vi "finish5PreparePassGamePlay.vi"(8 "error in (no error)":errorcluster, 9 "last_command":T1, 10 "Game":refnum<class "Game.lvclass">, 11 "5PreparePassGamePlay in":refnum<class "5PreparePassGamePlay.lvclass">) -> (0 "error out":errorcluster, 2 "result":bool, 3 "5PreparePassGamePlay out":refnum<class "5PreparePassGamePlay.lvclass">)   [LabVIEW 2020, in "5PreparePassGamePlay.lvclass"]
uses:
  5PreparePassGamePlay.lvclass
  Game_class/Game.lvclass
  Referee_class/command_interpreted.ctl
  Game_class/Game.lvclass/Game.ctl
  Referee_class/Referee.lvclass/Referee.ctl
  Referee_class/Read command_interpreted.vi
  Game_class/Read Referee.vi
  Game_class/Read TimeRef.vi
  Referee_class/Referee.lvclass
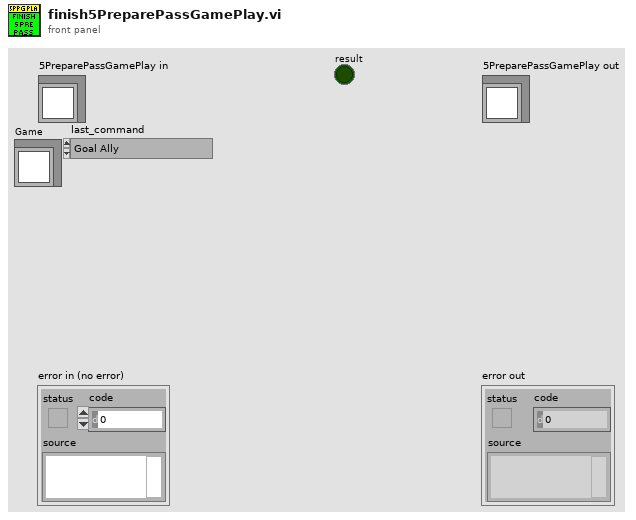
[diagram p1: front panel]
types:
  T1 = typedef "command_interpreted.ctl" = enum16{"Goal Ally", "Goal Enemy", "Ball Placement Enemy", "Ball Placement Ally", "Normal Half Time", "Extra Time  Break", "Extra Half Time", "None", "Post Game", "PKA Normal Start", "Prepare Kickoff Ally", "PKE Normal Start", "Prepare Kickoff Enemy", "Force Start", "Halt", "Timeout", "Prepare Penalty Ally", "Prepare Penalty Enemy", "PPA NormalStart", "PPE Normal Start", "Indirect Free Ally", "Direct Free Enemy", "Direct Free Ally", "Indirect Free Enemy", "Stop"}
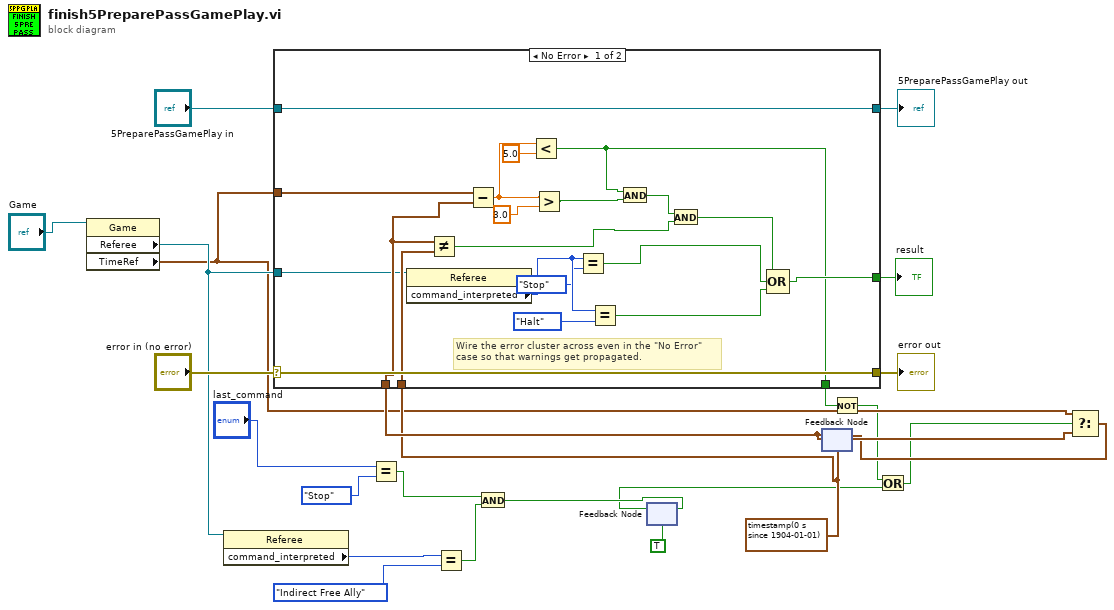
[diagram p0: block diagram]
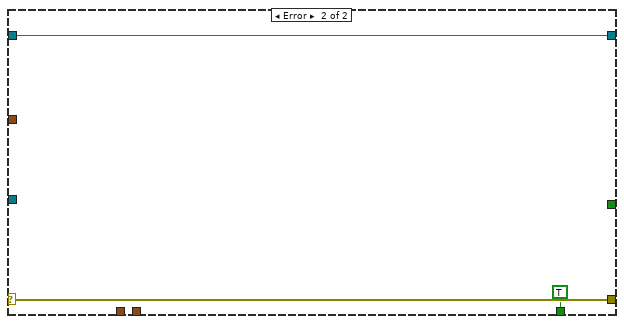
[diagram p2: hidden frame]
diagram:
  w8 = timestamp(0 s since 1904-01-01) ("TimeRef")
  n1 = property class="Game"(reference="Game") -> ("Referee"=w12:refnum<class "Referee.lvclass">, "TimeRef"=w7:timestamp)  [unwired: 1 in, 2 out]
  n2 = property class="Referee"(reference=w12) -> ("command_interpreted"=w15:T1)  [unwired: 1 in, 2 out]
  n3 = Equal?(x="last_command", y=command_interpreted."Stop") -> (x = y?=w10:bool)
  n4 = Equal?(x=w15, y=command_interpreted."Indirect Free Ally") -> (x = y?=w11:bool)
  n5 = And(x=w10, y=w11) -> (x .and. y?=w6:bool)
  n6 = feedback #1(TRUE) -> (w4:bool)
  n7 = feedback-in #1(w6) -> ()
  n8 = feedback #2(w8) -> (w18:timestamp)
  n9 = case shown="No Error" "error in (no error)" {
    selector: "error in (no error)" -> [w42 w46]
    tunnel: [w42 w46] -> w22
    tunnel: [w43 w45] -> w20
    tunnel: "5PreparePassGamePlay in" -> [w43 w45]
    tunnel: [w36 _] -> w19
    tunnel: w18 -> [w32 _]
    tunnel: w12 -> [w31 _]
    tunnel: w7 -> [w34 _]
    tunnel: w8 -> [w33 _]
    tunnel: [w24 TRUE] -> w2
    frame No Error {
      # "Wire the error cluster across even in the \"No Error\"\ncase so that warnings get propagated."
      n10 = property class="Referee"(reference=w31) -> ("command_interpreted"=w41:T1)  [unwired: 1 in, 2 out]
      n11 = Not Equal?(x=w32, y=w33) -> (x != y?=w27:bool)
      n12 = Subtract(x=w34, y=w32) -> (x-y=w30:dbl)
      n13 = Less?(x=w30, y=5.0) -> (x < y?=w24:bool)
      n14 = Greater?(x=w30, y=3.0) -> (0:w28:bool)
      n15 = Equal?(x=w41, y=command_interpreted."Stop") -> (x = y?=w37:bool)
      n16 = Equal?(x=w41, y=command_interpreted."Halt") -> (x = y?=w38:bool)
      n17 = And(x=w24, y=w28) -> (x .and. y?=w26:bool)
      n18 = And(x=w26, y=w27) -> (x .and. y?=w25:bool)
      n19 = Compound Arithmetic op=OR(w25, w37, w38) -> (w36:bool)
    }
    frame Error {
    }
  }
  "error out" <- w22
  "5PreparePassGamePlay out" <- w20
  "result" <- w19
  n20 = Not(x=w2) -> (.not. x?=w1:bool)
  n21 = Or(x=w1, y=w4) -> (x .or. y?=w3:bool)
  n22 = Select(t=w7, s=w3, f=w18) -> (s? t:f=w5:timestamp)
  n23 = feedback-in #2(w5) -> ()
